vi "Noise.vi"() -> (0 "White Noise Out":fxp<+/-,8,8> caption="Noise Out")   [LabVIEW 2015]
doc: "Generates an arbitrary sample in the range of [-128 , 127]."
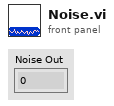
[diagram p1: front panel]
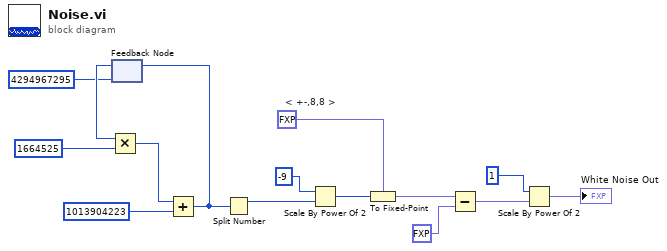
[diagram p0: block diagram]
diagram:
  w8 = fxp<+/-,8,8> 0.0  # < +-,8,8 >
  n1 = feedback #1(u32 4294967295 ("Seed")) -> (w12:u32)
  n2 = Multiply(x=w12, y=u32 1664525) -> (x*y=w15:u32)
  n3 = Add(x=w15, y=u32 1013904223 ("LCG constant C (add)")) -> (x+y=w10:u32)
  n4 = feedback-in #1(w10) -> ()
  n5 = Split Number(x=w10) -> (hi(x)=w7:u16)  [unwired: 1 out]
  n6 = Scale By Power Of 2(n=i8 -9 ("Uniform scale factor"), x=w7) -> (x*2^n=w3:u16)
  n7 = To Fixed-Point(fixed-point type=w8, number=w3) -> (fixed-point=w6:fxp<+/-,8,8>)
  n8 = Subtract(x=w6, y=fxp<+/-,8,8> 64.0) -> (x-y=w5:fxp<+/-,8,8>)
  n9 = Scale By Power Of 2(n=i16 1, x=w5) -> (x*2^n=→"White Noise Out":fxp<+/-,8,8>)
